vi "parse_config.vi"(11 "initial config":string="#define OFFSET_MAG_X 0.00\n#define OFFSET_MAG_Y 0.00\n#define OFFSET_MAG_Z 0.00\n#define R_MAG 1.00\n\n#define OFFSET_ACC_X 0.00\n#define OFFSET_ACC_Y 0.00\n#define OFFSET_ACC_Z 0.00\n#define R_ACC 1.00\n\n#define OFFSET_GYR_X 0.00\n#define OFFSET_GYR_Y 0.00\n#define OFFSET_GYR_Z 0.00") -> (3 "config":T2)   [LabVIEW 2019, in "Nano33BLE-TiltCompensationSupport.lvlib"]
uses:
  types/xyz.ctl
  <vilib>/regexp/Match Regular Expression.xnode
  Nano33BLE-TiltCompensationSupport.lvlib
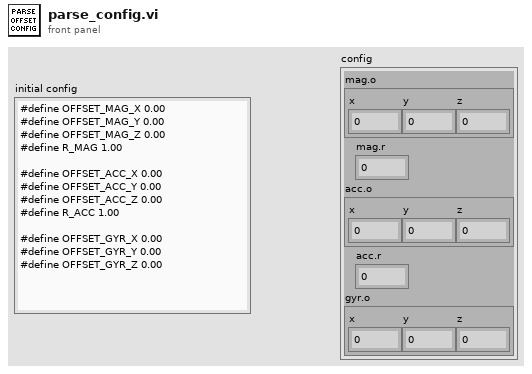
[diagram p1: front panel]
types:
  T1 = typedef "Nano33BLE-TiltCompensationSupport.lvlib/xyz.ctl" = cluster{"x":dbl, "y":dbl, "z":dbl}
  T2 = cluster{"mag.o":T1, "mag.r":dbl, "acc.o":T1, "acc.r":dbl, "gyr.o":T1}
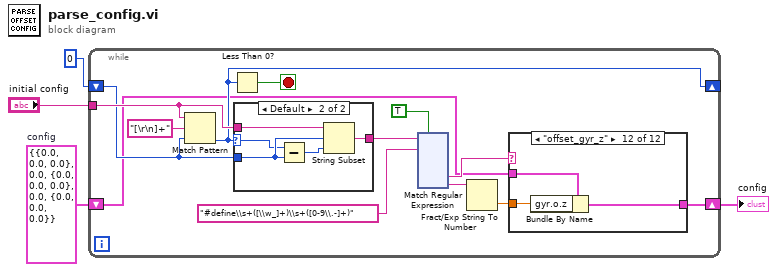
[diagram p0: block diagram]
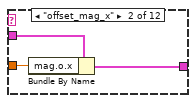
[diagram p3: hidden frame]
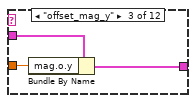
[diagram p4: hidden frame]
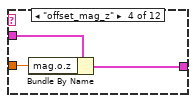
[diagram p5: hidden frame]
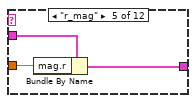
[diagram p6: hidden frame]
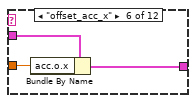
[diagram p7: hidden frame]
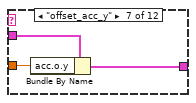
[diagram p8: hidden frame]
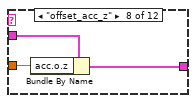
[diagram p9: hidden frame]
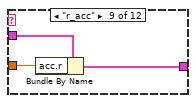
[diagram p10: hidden frame]
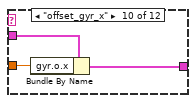
[diagram p11: hidden frame]
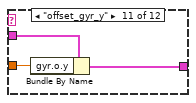
[diagram p12: hidden frame]
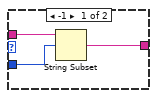
[diagram p13: hidden frame]
diagram:
  w2 = T2 {"mag.o"={"x"=0.0, "y"=0.0, "z"=0.0}, "mag.r"=0.0, "acc.o"={"x"=0.0, "y"=0.0, "z"=0.0}, "acc.r"=0.0, "gyr.o"={"x"=0.0, "y"=0.0, "z"=0.0}}  # config
  n1 = while {
    tunnel: "initial config" -> [w15]
    shift-right: [w13] -> _
    shift-left: 0 ("offset past match") -> [w14]
    shift-right: [w5] -> w1
    shift-left: w2 -> [w6]
    stop <- w16 stop-if-true
    n2 = Match Pattern(string=w15, regular expression="[\r\n]+", offset (0)=w14) -> (offset past match=w13:i32)  [unwired: 3 out]
    n3 = Less Than 0?(x=w13) -> (x < 0?=w16:bool)
    n4 = case shown="Default" w13 {
      selector: w13 -> [_ w174]
      tunnel: w15 -> [w171 w176]
      tunnel: w14 -> [w170 w175]
      tunnel: [w169 w172] -> w11
      frame -1 {
        n5 = String Subset(string=w171, offset (0)=w170) -> (substring=w169:string)  [unwired: 1 in]
      }
      frame Default {
        n6 = Subtract(x=w174, y=w175) -> (x-y=w173:i32)
        n7 = String Subset(string=w176, offset (0)=w175, length (rest)=w173) -> (substring=w172:string)
      }
    }
    n8 = xnode "Match Regular Expression"("input string"=w11, "regular expression"="#define\\s+([\\w_]+)\\s+([0-9\\.-]+)", "ignore case? (F)"=TRUE) -> ("submatch 1"=w9:string, "submatch 2"=w8:string)  [unwired: 3 in, 5 out]
    n9 = Fract/Exp String To Number(string=w8) -> (number=w7:dbl)  [unwired: 3 in, 1 out]
    n10 = case shown="\"offset_gyr_z\"" w9 {
      tunnel: w7 -> [_ w19 w22 w25 w28 w31 w34 w37 w40 w43 w46 w49]
      tunnel: w6 -> [w18 w21 w24 w27 w30 w33 w36 w39 w42 w45 w48 w51]
      tunnel: [w18 w20 w23 w26 w29 w32 w35 w38 w41 w44 w47 w50] -> w5
      frame Default {
      }
      frame "offset_mag_x" {
        n11 = Bundle By Name(cluster=w21, "mag.o.x"=w19) -> (w20:T2)
      }
      frame "offset_mag_y" {
        n12 = Bundle By Name(cluster=w24, "mag.o.y"=w22) -> (w23:T2)
      }
      frame "offset_mag_z" {
        n13 = Bundle By Name(cluster=w27, "mag.o.z"=w25) -> (w26:T2)
      }
      frame "r_mag" {
        n14 = Bundle By Name(cluster=w30, "mag.r"=w28) -> (w29:T2)
      }
      frame "offset_acc_x" {
        n15 = Bundle By Name(cluster=w33, "acc.o.x"=w31) -> (w32:T2)
      }
      frame "offset_acc_y" {
        n16 = Bundle By Name(cluster=w36, "acc.o.y"=w34) -> (w35:T2)
      }
      frame "offset_acc_z" {
        n17 = Bundle By Name(cluster=w39, "acc.o.z"=w37) -> (w38:T2)
      }
      frame "r_acc" {
        n18 = Bundle By Name(cluster=w42, "acc.r"=w40) -> (w41:T2)
      }
      frame "offset_gyr_x" {
        n19 = Bundle By Name(cluster=w45, "gyr.o.x"=w43) -> (w44:T2)
      }
      frame "offset_gyr_y" {
        n20 = Bundle By Name(cluster=w48, "gyr.o.y"=w46) -> (w47:T2)
      }
      frame "offset_gyr_z" {
        n21 = Bundle By Name(cluster=w51, "gyr.o.z"=w49) -> (w50:T2)
      }
    }
  }
  "config" <- w1
